vi "Read JSON File.vi"   [LabVIEW 2015, in "JSON.lvlib"]
uses:
  JSON.lvlib
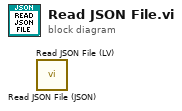
[diagram p0: block diagram]
diagram:
  n1 = call "Read JSON File (JSON).vi"() -> ()  [unwired: 10 in, 2 out]
  n2 = call "Read JSON File (LV).vi"() -> ()  [unwired: 10 in, 2 out]
